vi "Disconnect All Switches.vi"(8 "error in":errorcluster, 11 "File Path":path) -> (0 "error out":errorcluster)   [LabVIEW 2023]
uses:
  afd4346a-76eb-465e-8813-e5cb1ce8fd53.vi
  <vilib>/Utility/error.llb/Error Cluster From Error Code.vi
  <vilib>/Utility/file.llb/Read Delimited Spreadsheet (string).vi
  <vilib>/ErrorRing/Error Ring.xnode
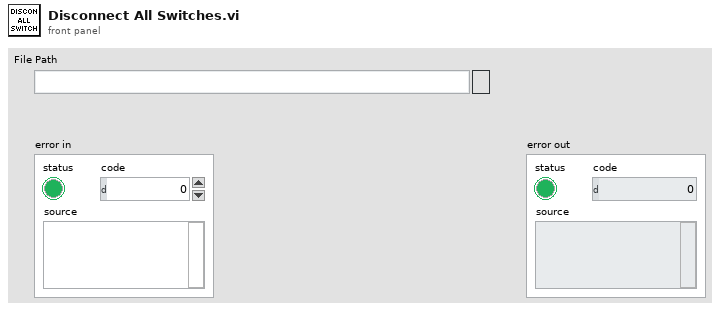
[diagram p1: front panel]
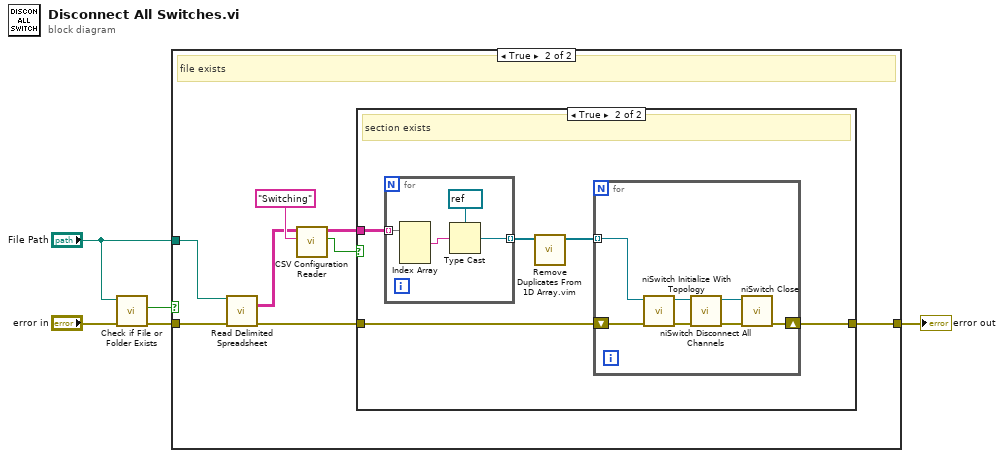
[diagram p0: block diagram]
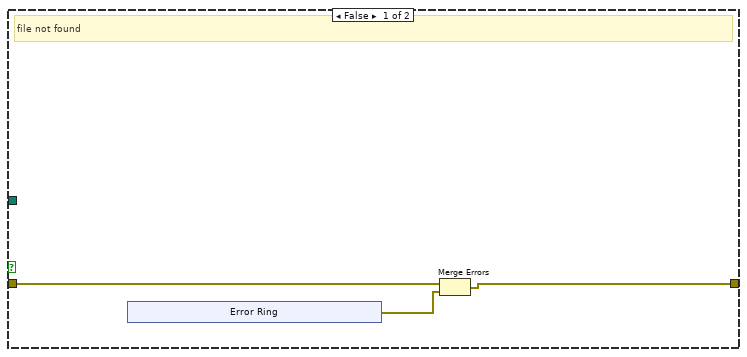
[diagram p2: hidden frame]
diagram:
  n1 = call <vilib>:"Check if File or Folder Exists.vi"("error in (no error)"="error in", "path"="File Path") -> ("error out"=w2:errorcluster, "file or folder exists?"=w4:bool)  [unwired: 7 in, 1 out]
  n2 = case shown="True" w4 {
    tunnel: "File Path" -> [_ w20]
    tunnel: [w8 w16] -> w1
    tunnel: w2 -> [w7 w15]
    frame False {
      # "file not found"
      n3 = xnode "Error Ring"() -> ("error out"=w6:errorcluster)
      n4 = Merge Errors(w7, w6) -> (w8:errorcluster)
    }
    frame True {
      # "file exists"
      n5 = call-poly <vilib>:"Read Delimited Spreadsheet.vi"("file path (dialog if empty)"=w20, "error in (no error)"=w15) -> ("all rows"=w18:string[][], "error out"=w14:errorcluster)  [unwired: 8 in, 4 out]
      n6 = call "CSV Configuration Reader.vi"("Section"="Switching" ("element"), "All CSV Configurations"=w18) -> ("Section Exists?"=w13:bool, "Extracted Configurations"=w17:string[][])  [unwired: 8 in]
      n7 = case shown="True" w13 {
        tunnel: w17 -> [_ w26]
        tunnel: [w21 w25] -> w16
        tunnel: w14 -> [w21 w24]
        frame False {
          # "section not found, no switching required"
        }
        frame True {
          # "section exists"
          n8 = for {
            tunnel: w26 -> [w37] mode=indexing
            tunnel: [w34] -> w23 mode=indexing
            n9 = Index Array(array=w37) -> (element #1=w36:string)  [unwired: 3 in, 2 out]
            n10 = Type Cast(type=refnum<k15> refnum ("Resource Name"), x=w36) -> (*(type *) &x=w34:refnum<k15>)
          }
          n11 = call "Remove Duplicates From 1D Array.vim"("array"=w23) -> ("array with duplicates removed"=w22:refnum<k15>[])  [unwired: 10 in]
          n12 = for {
            shift-right: [w31] -> w25
            shift-left: w24 -> [w30]
            tunnel: w22 -> [w29] mode=indexing
            n13 = call <instrlib>:"niSwitch Initialize With Topology.vi"("error in (no error)"=w30, "resource name"=w29) -> ("error out"=w32:errorcluster, "instrument handle out"=w33:refnum<k15>)  [unwired: 8 in]
            n14 = call <instrlib>:"niSwitch Disconnect All Channels.vi"("error in (no error)"=w32, "instrument handle"=w33) -> ("error out"=w28:errorcluster, "instrument handle out"=w27:refnum<k15>)  [unwired: 8 in]
            n15 = call <instrlib>:"niSwitch Close.vi"("error in (no error)"=w28, "instrument handle"=w27) -> ("error out"=w31:errorcluster)  [unwired: 9 in]
          }
        }
      }
    }
  }
  "error out" <- w1
